vi "switch request.vi"(8 "Num":u32[](array[numeric])=[1, 2, 3, 4], 9 "Z4_tmp(AutoSetState)":T1(array[ring])=[enum."stop ready", enum."stop ready", enum."stop ready", enum."stop ready"], 10 "Z3(State)":T1(array[ring])=[enum."stop ready", enum."stop ready", enum."stop ready", enum."stop ready"], 11 "Z1(CmdSource)":T2(array[ring])=[enum."auto", enum."auto", enum."auto", enum."auto"]) -> (0 "N off":i32, 1 "off request":bool[](array[boolean]), 2 "N on":i32, 3 "on request":bool[](array[boolean]), 4 "ok":bool[](array[boolean]))   [LabVIEW 2019, in "Userlib.lvlib"]
uses:
  Userlib.lvlib
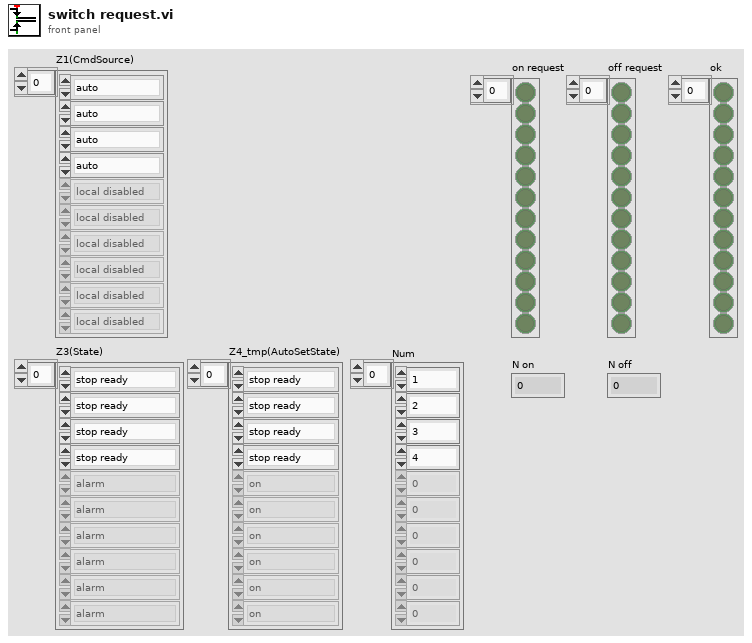
[diagram p1: front panel]
types:
  T1 = enum8{"alarm", "disabled", "not ready", "stop ready", "reserv", "switched off", "switched on", "check", "on min", "decrease speed", "on", "increase speed", "on max"}[]
  T2 = enum8{"local disabled", "local hand", "hand", "auto", "dist"}[]
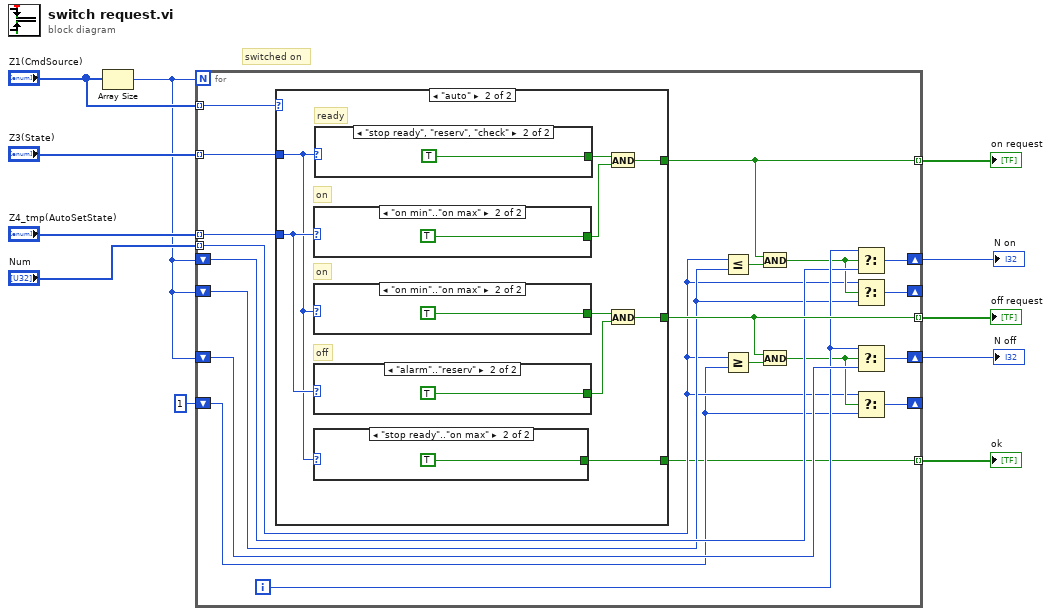
[diagram p0: block diagram]
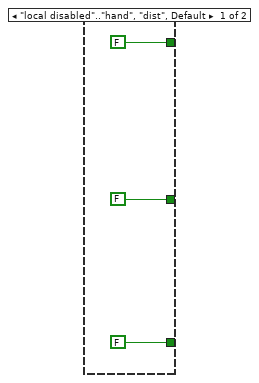
[diagram p2: hidden frame]
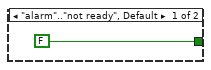
[diagram p3: hidden frame]
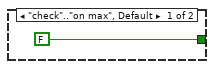
[diagram p4: hidden frame]
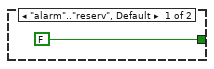
[diagram p5: hidden frame]
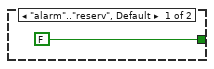
[diagram p6: hidden frame]
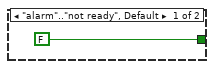
[diagram p7: hidden frame]
diagram:
  # "switched on"
  n1 = Array Size(array="Z1(CmdSource)") -> (size(s)=w3:i32)
  n2 = for {
    N: w3 -> [_]
    tunnel: "Z3(State)" -> [w31] mode=indexing
    tunnel: "Z1(CmdSource)" -> [w30] mode=indexing
    tunnel: "Z4_tmp(AutoSetState)" -> [w29] mode=indexing
    tunnel: [w27] -> w9 mode=indexing
    tunnel: [w23] -> w8 mode=indexing
    shift-right: [w20] -> w5
    shift-left: w3 -> [w21]
    shift-right: [w28] -> w7
    shift-left: w3 -> [w24]
    tunnel: "Num" -> [w15] mode=indexing
    shift-right: [w17] -> _
    shift-left: w3 -> [w18]
    shift-right: [w13] -> _
    shift-left: u32 1 ("Preset_state") -> [w14]
    tunnel: [w12] -> w1 mode=indexing
    i -> [w22]
    n3 = case shown="\"auto\"" w30 {
      tunnel: w31 -> [_ w36]
      tunnel: w29 -> [_ w37]
      tunnel: [FALSE w41] -> w27
      tunnel: [FALSE w38] -> w23
      tunnel: [FALSE w35] -> w12
      frame "local disabled".."hand", "dist", Default {
      }
      frame "auto" {
        # "off"
        # "on"
        # "on"
        # "ready"
        n4 = case shown="\"on min\"..\"on max\"" w37 {
          tunnel: [FALSE TRUE] -> w42
          frame "alarm".."reserv", Default {
          }
          frame "on min".."on max" {
          }
        }
        n5 = case shown="\"on min\"..\"on max\"" w36 {
          tunnel: [FALSE TRUE] -> w40
          frame "alarm".."reserv", Default {
          }
          frame "on min".."on max" {
          }
        }
        n6 = case shown="\"alarm\"..\"reserv\"" w37 {
          tunnel: [FALSE TRUE] -> w39
          frame "check".."on max", Default {
          }
          frame "alarm".."reserv" {
          }
        }
        n7 = case shown="\"stop ready\"..\"on max\"" w36 {
          tunnel: [FALSE TRUE] -> w35
          frame "alarm".."not ready", Default {
          }
          frame "stop ready".."on max" {
          }
        }
        n8 = case shown="\"stop ready\", \"reserv\", \"check\"" w36 {
          tunnel: [FALSE TRUE] -> w43
          frame "alarm".."not ready", Default {
          }
          frame "stop ready", "reserv", "check" {
          }
        }
        n9 = And(x=w43, y=w42) -> (x .and. y?=w41:bool)
        n10 = And(x=w40, y=w39) -> (x .and. y?=w38:bool)
      }
    }
    n11 = Less Or Equal?(x=w15, y=w18) -> (x <= y?=w26:bool)
    n12 = Greater Or Equal?(x=w15, y=w14) -> (x >= y?=w25:bool)
    n13 = And(x=w27, y=w26) -> (x .and. y?=w19:bool)
    n14 = And(x=w23, y=w25) -> (x .and. y?=w16:bool)
    n15 = Select(t=w22, s=w19, f=w21) -> (s? t:f=w20:i32)
    n16 = Select(t=w15, s=w19, f=w18) -> (s? t:f=w17:u32)
    n17 = Select(t=w22, s=w16, f=w24) -> (s? t:f=w28:i32)
    n18 = Select(t=w15, s=w16, f=w14) -> (s? t:f=w13:u32)
  }
  "on request" <- w9
  "off request" <- w8
  "N on" <- w5
  "N off" <- w7
  "ok" <- w1
